vi "Configure Red.vi"(8 "Error In":errorcluster, 11 "eCRDS in":refnum<class "eCRDS.lvclass">) -> (0 "error out":errorcluster, 3 "eCRDS out":refnum<class "eCRDS.lvclass">)   [LabVIEW 2014, in "eCRDS Library.lvlib" / "eCRDS.lvclass"]
doc: "Configure the red channel for generation and acquisition of the laser signal. The acquisition of the laser signal is run off of a retriggerable clock signal that operates in bursts. When the clock runs, a signal is acquired. The clock only runs when the digital output for the laser goes high. It then generates a finite number of signals until the laser output goes high again.\n\nThe clock for the AI runs off of the same board as the AI. The clock is triggered via a signal run across the backplane on PXI_Trig1 that is connected to the generation signal on the housekeeping card."
uses:
  eCRDS.lvclass
  eCRDS.lvclass/eCRDS.ctl
  reusable/Instrument/Instrument.lvclass/Instrument.ctl
  reusable/Instrument/Read Log Session.vi
  <vilib>/DAQmx/configure/timing.llb/DAQmx Timing (Implicit).vi
  <vilib>/DAQmx/configure/timing.llb/DAQmx Timing (Sample Clock).vi
  <userlib>/_Session Fwk/Session - Root.lvclass
  <resource>/objmgr/daqmx.rc
  reusable/Session APIs/Session Log/System Log.lvclass
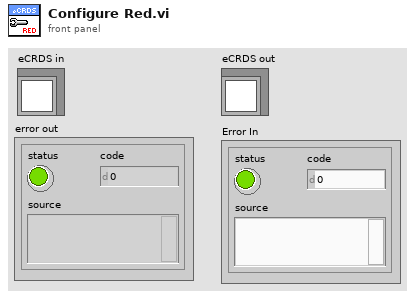
[diagram p1: front panel]
types:
  T1 = typedef "Session - Root.lvclass/Session Handle.ctl" = refnum<data-value>
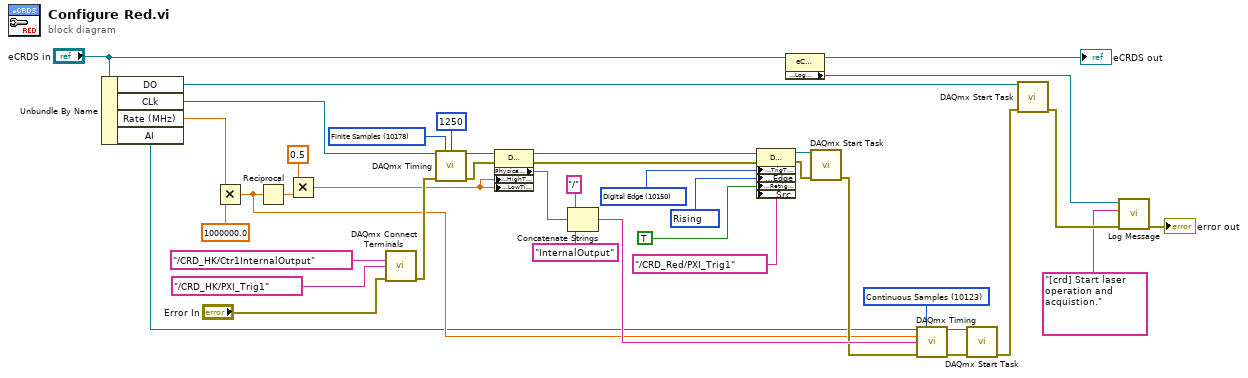
[diagram p0: block diagram]
diagram:
  w38 = 10123 items=["Finite Samples"=10178, "Continuous Samples"=10123, "Hardware Timed Single Point"=12522] ("sample mode")
  w26 = 10280 items=["Rising"=10280, "Falling"=10171] ("Ref.DigEdge.Edge")
  w25 = 10150 items=["Analog Edge"=10099, "Digital Edge"=10150, "Digital Pattern"=10398, "Analog Window"=10103, "None"=10230] ("Ref.TrigType")
  w17 = 10178 items=["Finite Samples"=10178, "Continuous Samples"=10123, "Hardware Timed Single Point"=12522] ("sample mode")
  n1 = Unbundle By Name("eCRDS in") -> ("DO"=w39:refnum<k21>, "CLk"=w16:refnum<k21>, "Rate (MHz)"=w13:dbl, "AI"=w8:refnum<k21>)
  n2 = Multiply(x=w13, y=1000000.0) -> (x*y=w12:dbl)
  n3 = Reciprocal(x=w12) -> (1/x=w11:dbl)
  n4 = Multiply(x=0.5, y=w11) -> (x*y=w9:dbl)
  n5 = call <vilib>:"DAQmx Connect Terminals.vi"("source terminal"=tag "/CRD_HK/Ctr1InternalOutput", "destination terminal"=tag "/CRD_HK/PXI_Trig1", "error in"="Error In") -> ("error out"=w35:errorcluster)  [unwired: 12 in]
  n6 = call-poly <vilib>:"DAQmx Timing.vi"("task/channels in"=w16, "sample mode"=w17, "samples per channel"=1250, "error in"=w35) -> ("task out"=w19:refnum<k21>, "error out"=w28:errorcluster)  [unwired: 10 in]
  n7 = property class="DAQmx Channel"(reference=w19, error in=w28, "CO.Pulse.HighTime"=w9, "CO.Pulse.LowTime"=w9) -> (reference out=w24:refnum<k21>, error out=w29:errorcluster, "PhysicalChanName"=w22:tag)
  n8 = Concatenate Strings("/" ("string"), w22, "InternalOutput" ("string")) -> (w23:string)
  n9 = property class="DAQmx Trigger"(reference=w24, error in=w29, "Start.TrigType"=w25, "Start.DigEdge.Edge"=w26, "Start.Retriggerable"=TRUE, "Start.DigEdge.Src"=tag "/CRD_Red/PXI_Trig1") -> (reference out=w30:refnum<k21>, error out=w31:errorcluster)
  n10 = property class="eCRDS"(reference="eCRDS in") -> (reference out=→"eCRDS out":refnum<class "eCRDS.lvclass">, "Accessors:Log Session"=w4:T1)  [unwired: 1 in, 1 out]
  n11 = call <vilib>:"DAQmx Start Task.vi"("task/channels in"=w30, "error in"=w31) -> ("error out"=w15:errorcluster)  [unwired: 12 in, 1 out]
  n12 = call-poly <vilib>:"DAQmx Timing.vi"("task/channels in"=w8, "sample mode"=w38, "rate"=w12, "source"=w23, "error in"=w15) -> ("task out"=w32:refnum<k21>, "error out"=w33:errorcluster)  [unwired: 9 in]
  n13 = call <vilib>:"DAQmx Start Task.vi"("task/channels in"=w32, "error in"=w33) -> ("error out"=w40:errorcluster)  [unwired: 12 in, 1 out]
  n14 = call <vilib>:"DAQmx Start Task.vi"("task/channels in"=w39, "error in"=w40) -> ("error out"=w3:errorcluster)  [unwired: 12 in, 1 out]
  n15 = call "Log Message.vi"("error in"=w3, "MSG In"="[crd] Start laser operation and acquistion.", "session in"=w4) -> ("error out"=→"error out":errorcluster)  [unwired: 7 in, 1 out]
